vi "Test VM Type.vi"() -> ()   [LabVIEW 2020]
uses:
  VoiceMeeterRemote/Voicemeeter Type.ctl
  VoiceMeeterRemote/VoiceMeeterRemote/VoiceMeeterRemote.lvclass
  VoiceMeeterRemote/VoiceMeeterRemote.lvlib
panel:
  out "Running?":bool
  out "Voicemeeter Type":T1=enum."Voicemeeter"
  out "error out":errorcluster
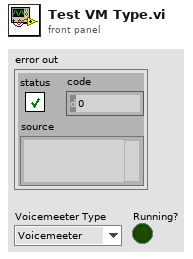
[diagram p1: front panel]
types:
  T1 = typedef "VoiceMeeterRemote.lvlib/Voicemeeter Type.ctl" = enum16{"Unknown", "Voicemeeter", "Banana", "Potato", "Potato x64"}
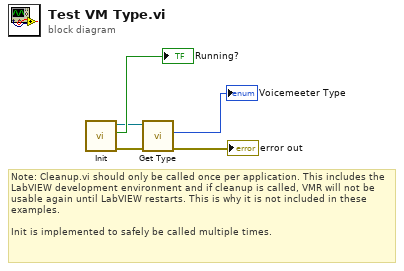
[diagram p0: block diagram]
diagram:
  # "Note: Cleanup.vi should only be called once per application. This includes the LabVIEW development environment and if cleanup is called, VMR will not be usable again until LabVIEW restarts. This is why it is not included in these examples.\n\nInit is implemented to safely be called multiple times."
  n1 = call "Init.vi"() -> ("error out"=w3:errorcluster, "Running?"=→"Running?":bool, "VoiceMeeterRemote out"=w4:refnum<class "VoiceMeeterRemote.lvclass">)  [unwired: 9 in]
  n2 = call "Get Type.vi"("error in (no error)"=w3, "VoiceMeeterRemote in"=w4) -> ("error out"=→"error out":errorcluster, "Type"=→"Voicemeeter Type":T1)  [unwired: 7 in, 1 out]
